vi "Get Array Configuration.vi"(8 "error in (no error)":errorcluster, 11 "Core Transfers Configuration in":refnum<class "Core Transfers Configuration.lvclass">) -> (0 "error out":errorcluster, 2 "transfer configurations":T1[](array[typedef]), 3 "Core Transfers Configuration out":refnum<class "Core Transfers Configuration.lvclass">)   [LabVIEW 2017, in "DSF Core.lvlib" / "Core Transfers Configuration.lvclass"]
uses:
  Core Transfers Configuration.lvclass
  Configuration.ctl
  Core Transfers Configuration.lvclass/Core Transfers Configuration.ctl
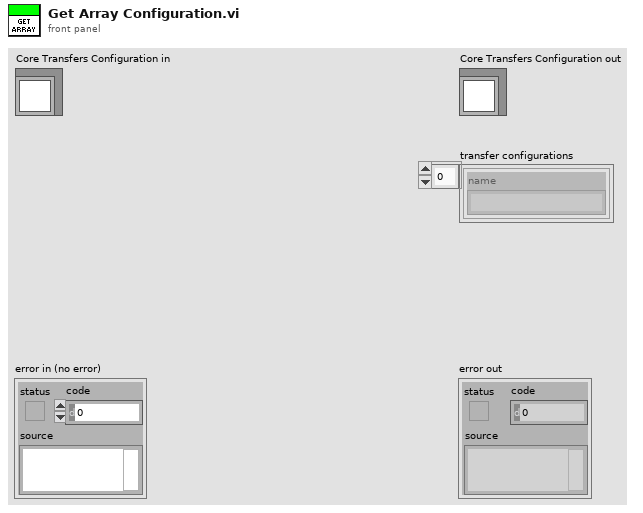
[diagram p1: front panel]
types:
  T1 = typedef "DSF Core.lvlib/Core Transfers Configuration.lvclass/Configuration.ctl" = cluster{"name":string}
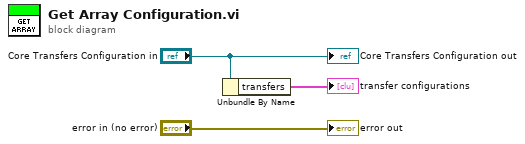
[diagram p0: block diagram]
diagram:
  n1 = Unbundle By Name("Core Transfers Configuration in") -> ("transfers"=→"transfer configurations":T1[])
  "error out" <- "error in (no error)"
  "Core Transfers Configuration out" <- "Core Transfers Configuration in"
